vi "Get Step Timing.vi"(8 "error in (no error)":errorcluster, 9 "Wash Step":T1, 10 "Vehicle Position":T2, 11 "Car Wash Controller in":refnum<class "Car Wash Controller.lvclass">) -> (0 "error out":errorcluster, 2 "Step Timing":dbl, 3 "Car Wash Controller out":refnum<class "Car Wash Controller.lvclass">)   [LabVIEW 2012, in "Car Wash Controller.lvlib" / "Car Wash Controller.lvclass"]
uses:
  Car Wash Controller.lvclass
  Vehicle Position.ctl
  Wash Step.ctl
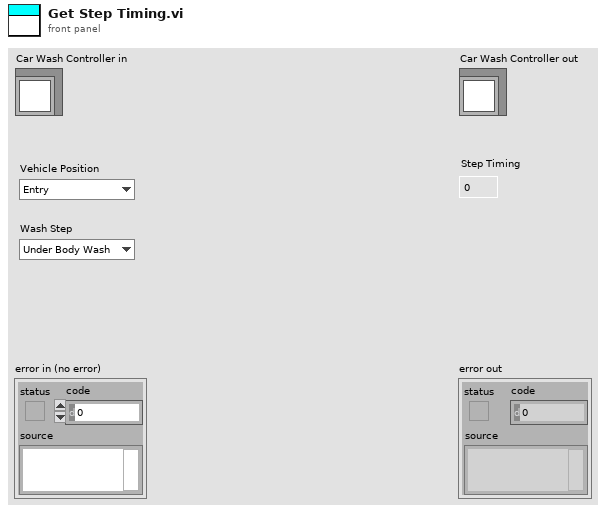
[diagram p1: front panel]
types:
  T1 = typedef "Car Wash Controller.lvlib/Car Wash Controller.lvclass/Wash Step.ctl" = enum16{"Under Body Wash", "Bug Remover", "Pre-Soak", "High Pressure Wash", "Low Pressure Wax", "Spot Free Rince", "Tire Shine Foam", "Air Dry"}
  T2 = typedef "Car Wash Controller.lvlib/Car Wash Controller.lvclass/Vehicle Position.ctl" = enum16{"Entry", "Station 1", "Station 2", "Station 3", "Exit"}
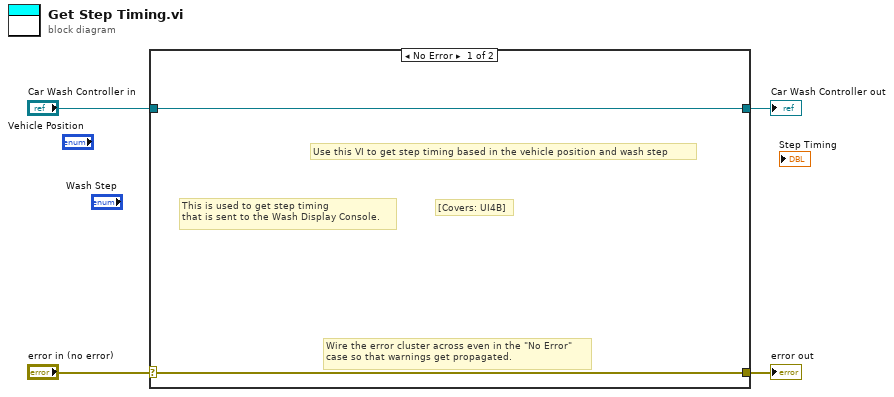
[diagram p0: block diagram]
diagram:
  n1 = case shown="No Error" "error in (no error)" {
    selector: "error in (no error)" -> [w5 w8]
    tunnel: [w5 w8] -> w3
    tunnel: [w6 w7] -> w1
    tunnel: "Car Wash Controller in" -> [w6 w7]
    frame No Error {
      # "This is used to get step timing\nthat is sent to the Wash Display Console."
      # "[Covers: UI4B]"
      # "Use this VI to get step timing based in the vehicle position and wash step"
      # "Wire the error cluster across even in the \"No Error\"\ncase so that warnings get propagated."
    }
    frame Error {
    }
  }
  "error out" <- w3
  "Car Wash Controller out" <- w1
